vi "Actor Core.vi"(8 "error in":errorcluster, 11 "Create Project View in":refnum<class "Create Project View.lvclass">) -> (0 "error out":errorcluster, 3 "Actor out":refnum<class "Actor.lvclass">)   [LabVIEW 2013, in "Create Project View.lvlib" / "Create Project View.lvclass"]
doc: "(<B>Filename</B>: Actor Framework.lvlib:Actor.lvclass:Actor Core.vi)\n\nReceives messages to the actor, reacts to them, and initiates any error handling that may shut the actor down.\n\nDescendant classes may override this VI to append parallel tasks for the actor to complete while it handles messages. Overrides use the Call Parent Method node."
uses:
  Create Project View.lvclass
  <vilib>/ActorFramework/Actor/Actor.lvclass
  Resources/UI Controls/Common/Side Button.ctl
  <vilib>/ActorFramework/Actor/Actor.lvclass/Actor.ctl
  <vilib>/ActorFrameworkMVC/View Actor/View Actor.lvclass
  <vilib>/ActorFramework/Message Enqueuer/Message Enqueuer.lvclass/Message Enqueuer.ctl
  Create Project View.lvclass/Create Project View.ctl
  <vilib>/Utility/miscctls.llb/LVPositionTypeDef.ctl
  Models/Create Project Model Messages/Set Item Configurations Msg/Set Item Configurations Msg.lvclass/Set Item Configurations Msg.ctl
  <vilib>/ActorFrameworkMVC/UI Controller Messages/Move Subpanel Msg/Move Subpanel Msg.lvclass/Move Subpanel Msg.ctl
  <vilib>/ActorFrameworkMVC/UI Controller Messages/Insert Subpanel Msg/Insert Subpanel Msg.lvclass/Insert Subpanel Msg.ctl
  <vilib>/ActorFramework/Message Enqueuer/Init from Existing Queue.vi
  <vilib>/ActorFramework/Message Enqueuer/Enqueue.vi
  <vilib>/ActorFramework/Message Priority Queue/Priority Enqueue.vi
  <vilib>/ActorFramework/Message Enqueuer/Message Enqueuer.lvclass
  Models/Create Project Model Messages/Set Item Configurations Msg/Set Item Configurations Msg.lvclass
  Models/Create Project Model Messages/Create Project Msg/Create Project Msg.lvclass
  <vilib>/ActorFrameworkMVC/UI Controller Messages/Move Subpanel Msg/Move Subpanel Msg.lvclass
  <vilib>/ActorFrameworkMVC/UI Controller Messages/Insert Subpanel Msg/Insert Subpanel Msg.lvclass
  Models/Project Model Messages/Preview Project Msg/Preview Project Msg.lvclass
  Models/Project Model Messages/Update Tiles Info Msg/Update Tiles Info Msg.lvclass
  Models/Project Model Messages/Update Previous Button Visibility Msg/Update Previous Button Visibility Msg.lvclass
  Models/Project Model Messages/Update Next Button Visibility Msg/Update Next Button Visibility Msg.lvclass
  Common/File IO/File IO.lvlib
  <vilib>/ActorFrameworkMVC/UI Controller Messages/Get Model Actor Enqueuer Msg/Get Model Actor Enqueuer Msg.lvclass
  <vilib>/ActorFrameworkMVC/View Actor Messages/Get Model Enqueuer Msg/Get Model Enqueuer Msg.lvclass
  Resources/UI Controls/UI Control.lvlib
panel:
  in  "Cancel":bool
  in  "Save":bool
  out "Tab Control":T1(tab)
  in  "Project Tester":string caption="项目检测人员："
  in  "Project Date":timestamp caption="项目日期：" format="%<%x>T"
  in  "Project Description":string caption="项目描述："
  in  "Project Name":string caption="项目名称："
  in  "Completion Date":timestamp caption="竣工日期：" format="%<%x>T"
  in  "CC Principal Telephone":string caption="联系电话："
  in  "CC Principal":string caption="负责人："
  in  "Construction Committee":string caption="主管建委："
  in  "Principal Telephone":string caption="联系电话："
  in  "Principal":string caption="负责人："
  in  "Communication Address":string caption="通讯地址："
  in  "Identification Level":u16(ring) caption="标识等级："
  in  "Identification Type":u16(ring) caption="标识类别："
  in  "Building Area":string caption="建筑面积："
  in  "Climate Classification":u16(ring) caption="气候分区："
  in  "Project Type":u16(ring) caption="工程类别："
  in  "Project Province":u16(ring) caption="项目地点："
  in  "Project City":u16(ring)
  in  "Project Address":string caption="详细地址："
  in  "Building Type":u16(ring) caption="建筑类型："
  in  "Construction Unit":string caption="建设单位："
  in  "Construction Date":timestamp caption="建设日期：" format="%<%x>T"
  in  "Spec 16":string caption="可再利用材料使用率（%）"
  in  "Spec 15":string caption="可再利用材料重量（t）"
  in  "Spec 14":string caption="可再循环材料利用率（%）"
  in  "Spec 13":string caption="可循环材料重量（t）"
  in  "Spec 12":string caption="建筑材料总重量（t）"
  in  "Spec 11":string caption="非传统水资源利用率（%）"
  in  "Spec 10":string caption="总用水量（m3/a）"
  in  "Spec 9":string caption="非传统水量（m3/a）"
  in  "Spec 8":string caption="节能率（%）"
  in  "Spec 7":string caption="单位面积能耗（kW-H/(m2a)）"
  in  "Spec 6":string caption="建筑总能耗（MJ/a）"
  in  "Spec 5":string caption="透水地面面积比（%）"
  in  "Spec 4":string caption="地下面积比（%）"
  in  "Spec 3":string caption="地下建筑面积（m2）"
  in  "Spec 2":string caption="建筑总面积（万m2）"
  in  "Spec 1":string caption="用地面积（万m2）"
  in  "Side Buttons":T1(radio)
  # "新建项目"
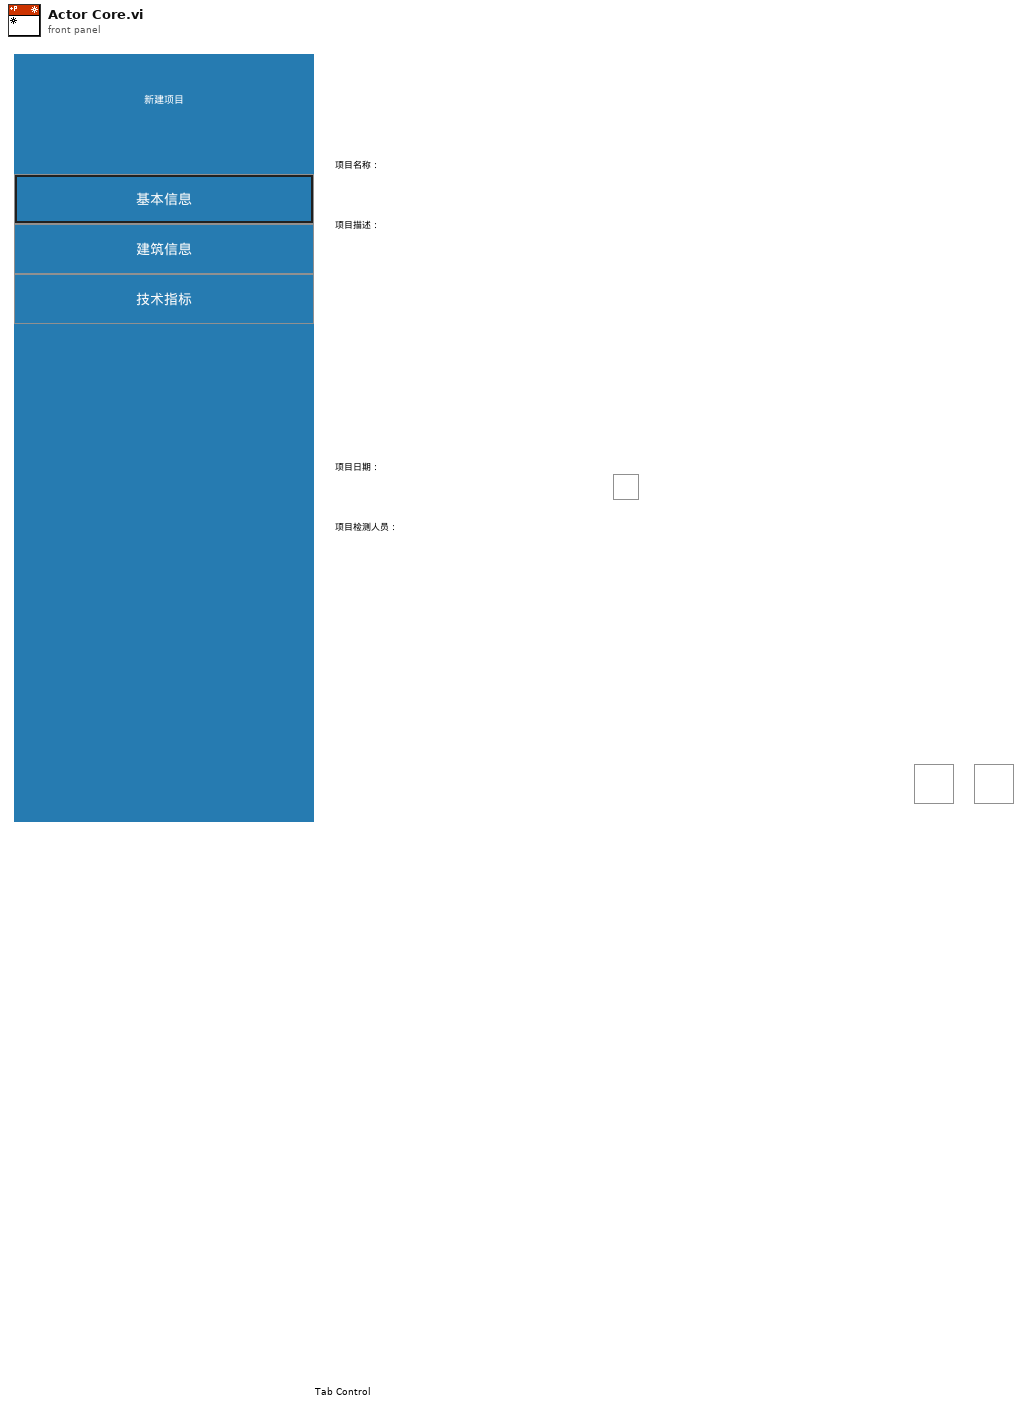
[diagram p1: front panel]
types:
  T1 = enum32{"Basic Info", "Building Info", "Specification"}
  T2 = typedef "Create Project View.lvlib/Create Project View.lvclass/Events.ctl" = cluster{"Reinitialize All":refnum<user-event>, "Key Focus":refnum<user-event>}
  T3 = typedef "LVPositionTypeDef.ctl" = cluster{"Left":i32, "Top":i32}
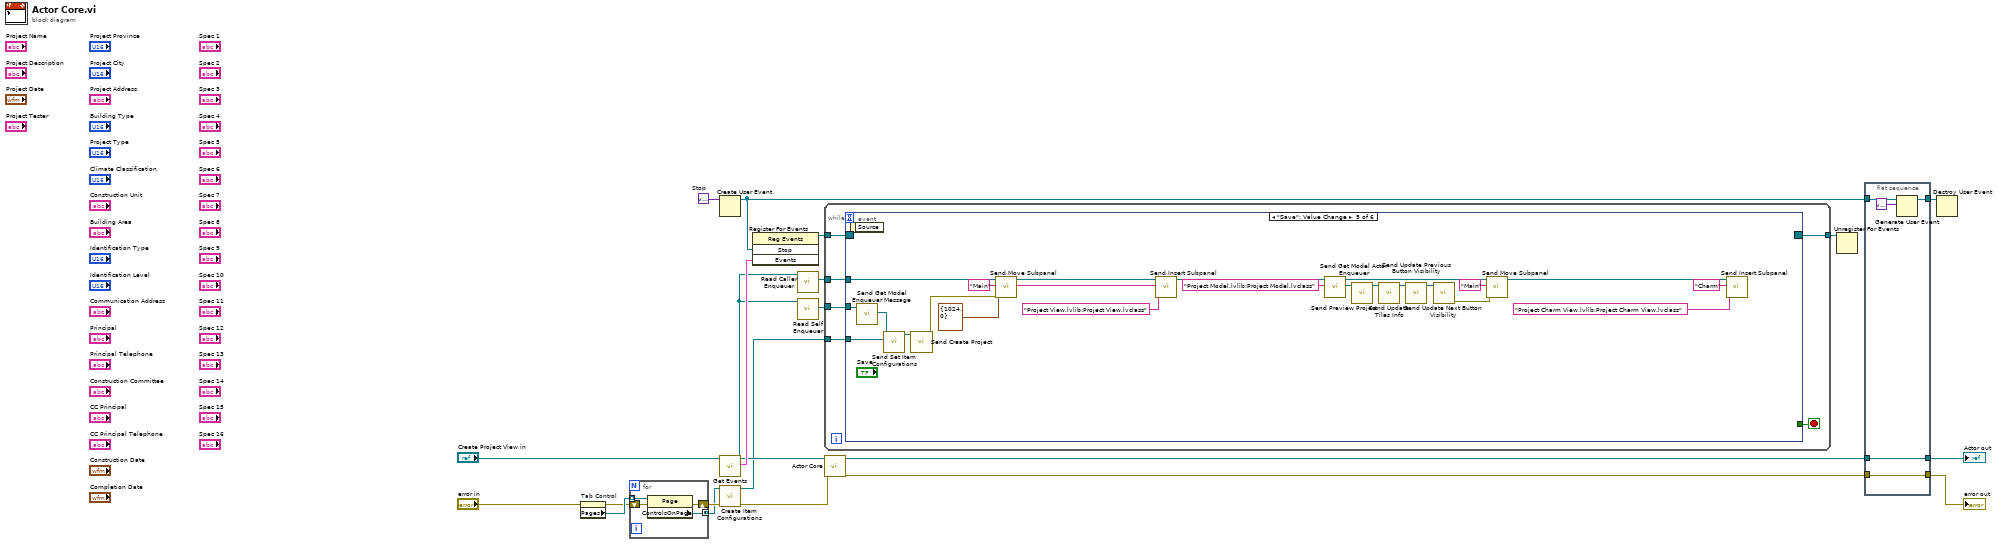
[diagram p0: block diagram]
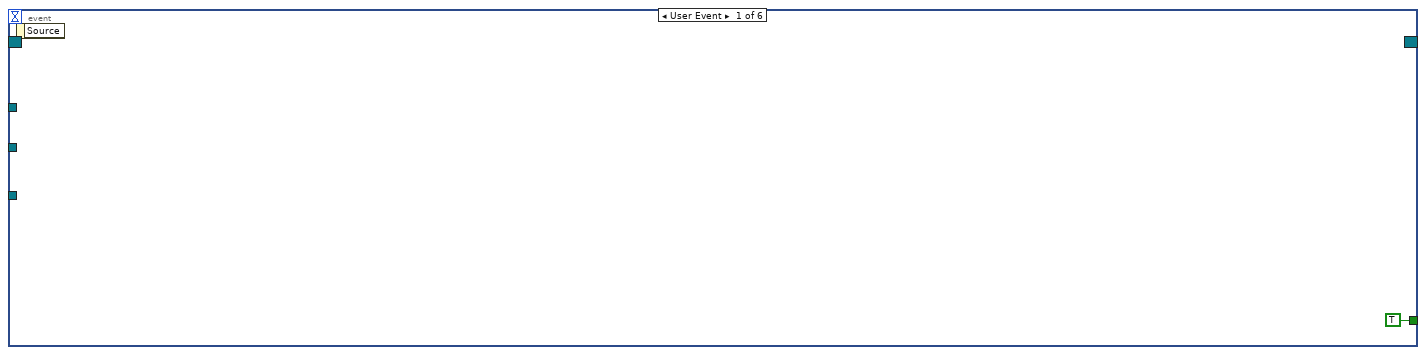
[diagram p2: hidden frame]
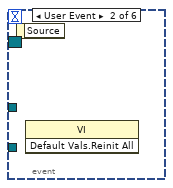
[diagram p3: hidden frame]
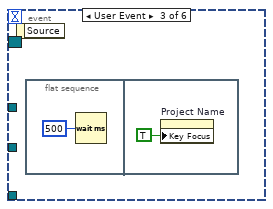
[diagram p4: hidden frame]
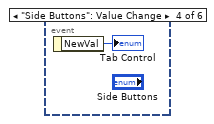
[diagram p5: hidden frame]
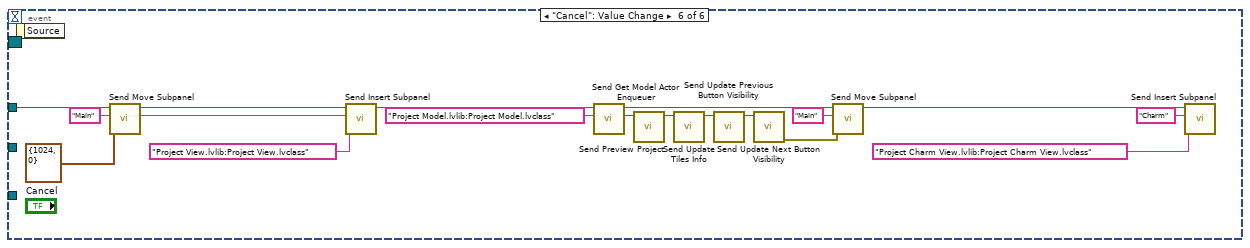
[diagram p6: hidden frame]
diagram:
  w21 = variant  # Stop
  n1 = property on="Tab Control" class="TabCtl (strict)"(error in="error in") -> (error out=w9:errorcluster, "Pages"=w10:refnum<vi>[])  [unwired: 1 in, 1 out]
  n2 = for {
    tunnel: w10 -> [w25] mode=indexing
    tunnel: [w24] -> w5 mode=concatenating
    shift-right: [w22] -> w7
    shift-left: w9 -> [w23]
    n3 = property class="Page"(reference=w25, error in=w23) -> (error out=w22:errorcluster, "ControlsOnPage"=w24:refnum<vi>[])  [unwired: 1 out]
  }
  n4 = Create User Event(user event datatype=w21) -> (user event=w13:refnum<user-event>)  [unwired: 1 in, 1 out]
  n5 = call "Get Events.vi"("Create Project View in"="Create Project View in") -> ("Events"=w12:T2, "Create Project View out"=w3:refnum<class "Create Project View.lvclass">)  [unwired: 9 in]
  n6 = call "Create Item Configurations.vi"("error in (no error)"=w7, "Controls References"=w5) -> ("error out"=w6:errorcluster, "Item Configurations"=w1:refnum<class "Item Configuration.lvclass">[])  [unwired: 8 in]
  n7 = register-events(w13, w12) -> (reference out=w14:refnum<event-registration>)  [unwired: 2 in, 1 out]
  n8 = call <vilib>:"Read Caller Enqueuer.vi"("Actor"=w3) -> ("Caller Enqueuer"=w4:refnum<class "Message Enqueuer.lvclass">)  [unwired: 10 in]
  n9 = call <vilib>:"Read Self Enqueuer.vi"("Actor"=w3) -> ("Self Enqueuer"=w2:refnum<class "Message Enqueuer.lvclass">)  [unwired: 10 in]
  n10 = while {
    tunnel: [w31] -> w11
    tunnel: w14 -> [w29]
    tunnel: w4 -> [w28]
    tunnel: w2 -> [w27]
    tunnel: w1 -> [w26]
    stop <- w30 stop-if-true
    n11 = event shown="[4] \"Save\": Value Change" {
      selector: w29 -> [_ _ _ _ _ _]
      dyn-events: [_ _ _ _ _ _] -> w31
      timeout: _ -> [_ _ _ _ _ _]
      tunnel: [TRUE _ _ _ _ _] -> w30
      tunnel: w28 -> [_ _ _ _ w37 w59]
      tunnel: w27 -> [_ _ _ _ w40 _]
      tunnel: w26 -> [_ _ _ _ w38 _]
      event User Event {
        n12 = event-data() -> ()  [unwired: 1 in, 1 out]
      }
      event User Event {
        n13 = event-data() -> ()  [unwired: 1 in, 1 out]
        n14 = invoke class="VI" method="Default Vals.Reinit All"() -> ()  [unwired: 3 in, 3 out]
      }
      event User Event {
        n15 = event-data() -> ()  [unwired: 1 in, 1 out]
        n16 = flat-sequence {
          frame #0 {
            n17 = Wait (ms)(milliseconds to wait=u32 500) -> ()  [unwired: 1 out]
          }
          frame #1 {
            n18 = property on="Project Name" class="Str"("Key Focus"=TRUE) -> ()  [unwired: 2 in, 2 out]
          }
        }
      }
      event "Side Buttons": Value Change {
        n19 = event-data() -> ("NewVal"=→"Tab Control":T1)  [unwired: 1 in]
      }
      event "Save": Value Change {
        w54 = "Main" ("Subpanel Name")
        n20 = event-data() -> ()  [unwired: 1 in, 1 out]
        n21 = call <vilib>:"Send Get Model Enqueuer Message.vi"("Message Enqueuer in"=w40) -> ("Reply"=w41:refnum<class "Message Enqueuer.lvclass">)  [unwired: 7 in, 3 out]
        n22 = call "Send Set Item Configurations.vi"("Item Configurations"=w38, "Message Enqueuer"=w41) -> ("Message Enqueuer out"=w39:refnum<class "Message Enqueuer.lvclass">)  [unwired: 8 in, 1 out]
        n23 = call "Send Create Project.vi"("Message Enqueuer"=w39) -> ("error out"=w42:errorcluster)  [unwired: 9 in, 1 out]
        n24 = call <vilib>:"Send Move Subpanel.vi"("error in (no error)"=w42, "Position (0,0)"=T3 {"Left"=1024, "Top"=0}, "Subpanel Name"=w54, "Message Enqueuer"=w37) -> ("Message Enqueuer out"=w57:refnum<class "Message Enqueuer.lvclass">)  [unwired: 6 in, 1 out]
        n25 = call <vilib>:"Send Insert Subpanel.vi"("View Name"="Project View.lvlib:Project View.lvclass" ("Subpanel Name"), "Subpanel Name"=w54, "Message Enqueuer"=w57) -> ("Message Enqueuer out"=w51:refnum<class "Message Enqueuer.lvclass">)  [unwired: 7 in, 1 out]
        n26 = call <vilib>:"Send Get Model Actor Enqueuer.vi"("Model Name"="Project Model.lvlib:Project Model.lvclass", "Message Enqueuer in"=w51) -> ("Reply"=w36:refnum<class "Message Enqueuer.lvclass">, "Message Enqueuer out"=w50:refnum<class "Message Enqueuer.lvclass">)  [unwired: 6 in, 2 out]
        n27 = call "Send Preview Project.vi"("Message Enqueuer"=w36) -> ("Message Enqueuer out"=w52:refnum<class "Message Enqueuer.lvclass">)  [unwired: 9 in, 1 out]
        n28 = call "Send Update Tiles Info.vi"("Message Enqueuer"=w52) -> ("Message Enqueuer out"=w48:refnum<class "Message Enqueuer.lvclass">)  [unwired: 9 in, 1 out]
        n29 = call "Send Update Previous Button Visibility.vi"("Message Enqueuer"=w48) -> ("Message Enqueuer out"=w47:refnum<class "Message Enqueuer.lvclass">)  [unwired: 9 in, 1 out]
        n30 = call "Send Update Next Button Visibility.vi"("Message Enqueuer"=w47) -> ("error out"=w46:errorcluster)  [unwired: 9 in, 1 out]
        n31 = call <vilib>:"Send Move Subpanel.vi"("error in (no error)"=w46, "Subpanel Name"="Main", "Message Enqueuer"=w50) -> ("Message Enqueuer out"=w45:refnum<class "Message Enqueuer.lvclass">)  [unwired: 7 in, 1 out]
        n32 = call <vilib>:"Send Insert Subpanel.vi"("View Name"="Project Charm View.lvlib:Project Charm View.lvclass", "Subpanel Name"="Charm", "Message Enqueuer"=w45) -> ()  [unwired: 7 in, 2 out]
      }
      event "Cancel": Value Change {
        w71 = "Main" ("Subpanel Name")
        n33 = event-data() -> ()  [unwired: 1 in, 1 out]
        n34 = call <vilib>:"Send Move Subpanel.vi"("Position (0,0)"=T3 {"Left"=1024, "Top"=0}, "Subpanel Name"=w71, "Message Enqueuer"=w59) -> ("Message Enqueuer out"=w74:refnum<class "Message Enqueuer.lvclass">)  [unwired: 7 in, 1 out]
        n35 = call <vilib>:"Send Insert Subpanel.vi"("View Name"="Project View.lvlib:Project View.lvclass" ("Subpanel Name"), "Subpanel Name"=w71, "Message Enqueuer"=w74) -> ("Message Enqueuer out"=w68:refnum<class "Message Enqueuer.lvclass">)  [unwired: 7 in, 1 out]
        n36 = call <vilib>:"Send Get Model Actor Enqueuer.vi"("Model Name"="Project Model.lvlib:Project Model.lvclass", "Message Enqueuer in"=w68) -> ("Reply"=w58:refnum<class "Message Enqueuer.lvclass">, "Message Enqueuer out"=w67:refnum<class "Message Enqueuer.lvclass">)  [unwired: 6 in, 2 out]
        n37 = call "Send Preview Project.vi"("Message Enqueuer"=w58) -> ("Message Enqueuer out"=w69:refnum<class "Message Enqueuer.lvclass">)  [unwired: 9 in, 1 out]
        n38 = call "Send Update Tiles Info.vi"("Message Enqueuer"=w69) -> ("Message Enqueuer out"=w65:refnum<class "Message Enqueuer.lvclass">)  [unwired: 9 in, 1 out]
        n39 = call "Send Update Previous Button Visibility.vi"("Message Enqueuer"=w65) -> ("Message Enqueuer out"=w64:refnum<class "Message Enqueuer.lvclass">)  [unwired: 9 in, 1 out]
        n40 = call "Send Update Next Button Visibility.vi"("Message Enqueuer"=w64) -> ("error out"=w63:errorcluster)  [unwired: 9 in, 1 out]
        n41 = call <vilib>:"Send Move Subpanel.vi"("error in (no error)"=w63, "Subpanel Name"="Main", "Message Enqueuer"=w67) -> ("Message Enqueuer out"=w62:refnum<class "Message Enqueuer.lvclass">)  [unwired: 7 in, 1 out]
        n42 = call <vilib>:"Send Insert Subpanel.vi"("View Name"="Project Charm View.lvlib:Project Charm View.lvclass", "Subpanel Name"="Charm", "Message Enqueuer"=w62) -> ()  [unwired: 7 in, 2 out]
      }
    }
  }
  n43 = call-parent "Actor Core.vi"("error in"=w6, "View Actor in"=w3) -> ("error out"=w17:errorcluster, "Actor out"=w18:refnum<class "Actor.lvclass">)  [unwired: 8 in]
  n44 = Unregister For Events(event registration refnum=w11) -> ()  [unwired: 1 in, 1 out]
  n45 = flat-sequence "Generate a stop event when the actor core stopped." {
    tunnel: w13 -> [w79]
    tunnel: [w77] -> w20
    tunnel: w18 -> [w76]
    tunnel: w17 -> [w75]
    tunnel: [w76] -> w16
    tunnel: [w75] -> w15
    frame #0 {
      n46 = Generate User Event(user event=w79, event data cluster=variant ("event data")) -> (user event out=w77:refnum<user-event>)  [unwired: 2 in, 1 out]
    }
  }
  n47 = Destroy User Event(user event=w20) -> ()  [unwired: 1 in, 1 out]
  "error out" <- w15
  "Actor out" <- w16
